vi "rsscope Query OPC.vi"(8 "error in (no error)":errorcluster, 11 "VISA resource name":refnum<visa-resource-name>) -> (0 "error out":errorcluster, 2 "OPC":i32, 3 "VISA resource name out":refnum<visa-resource-name>)   [LabVIEW 2014]
doc: "This VI sends OPC query to the instrument. This effectively causes your program to wait in this VI until the instrument has processed all the commands you have sent to it until this point. Use the VI to force the synchronization of the instrument with you program.\n\nAttribute:\n-\n\nRemote-control command:\n*OPC?"
uses:
  _utility/rsidr_core.llb/rsscope_rsidr_core.lvlib
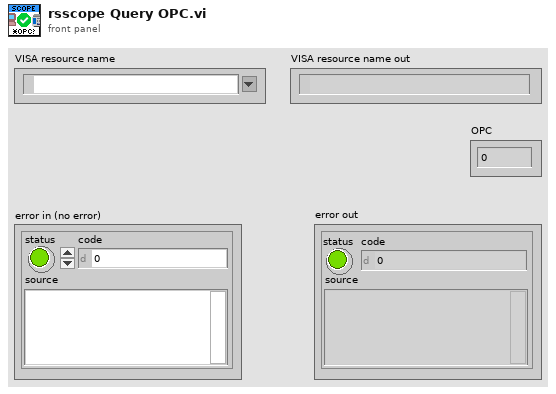
[diagram p1: front panel]
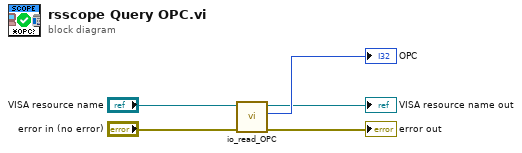
[diagram p0: block diagram]
diagram:
  n1 = call "io_read_OPC.vi"("error in"="error in (no error)", "VISA resource name"="VISA resource name") -> ("error out"=→"error out":errorcluster, "OPC returned"=→"OPC":i32, "VISA resource name out"=→"VISA resource name out":refnum<visa-resource-name>)  [unwired: 7 in]
